vi "AnalogAQ Canales.vi"(8 "error in":errorcluster, 9 "Numero de Muestras":i32=1000, 10 "Frecuencia":dbl=1000.0 format="%0.2f", 11 "Canales":tag[](array[tag])) -> (0 "error out":errorcluster, 3 "Classic DAQmx Task Name":refnum<k21>)   [LabVIEW 2020]
uses:
  <vilib>/DAQmx/create/channels.llb/DAQmx Create Channel (AI-Voltage-Basic).vi
  <vilib>/DAQmx/configure/timing.llb/DAQmx Timing (Sample Clock).vi
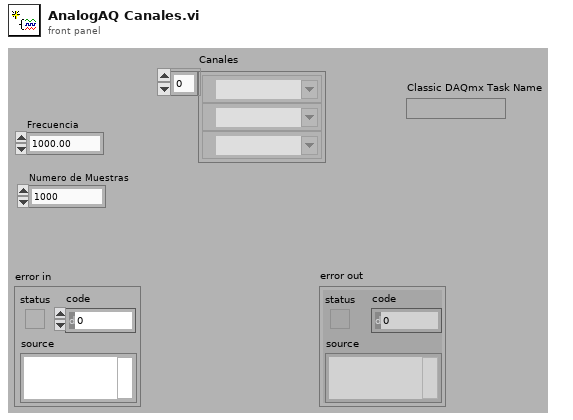
[diagram p1: front panel]
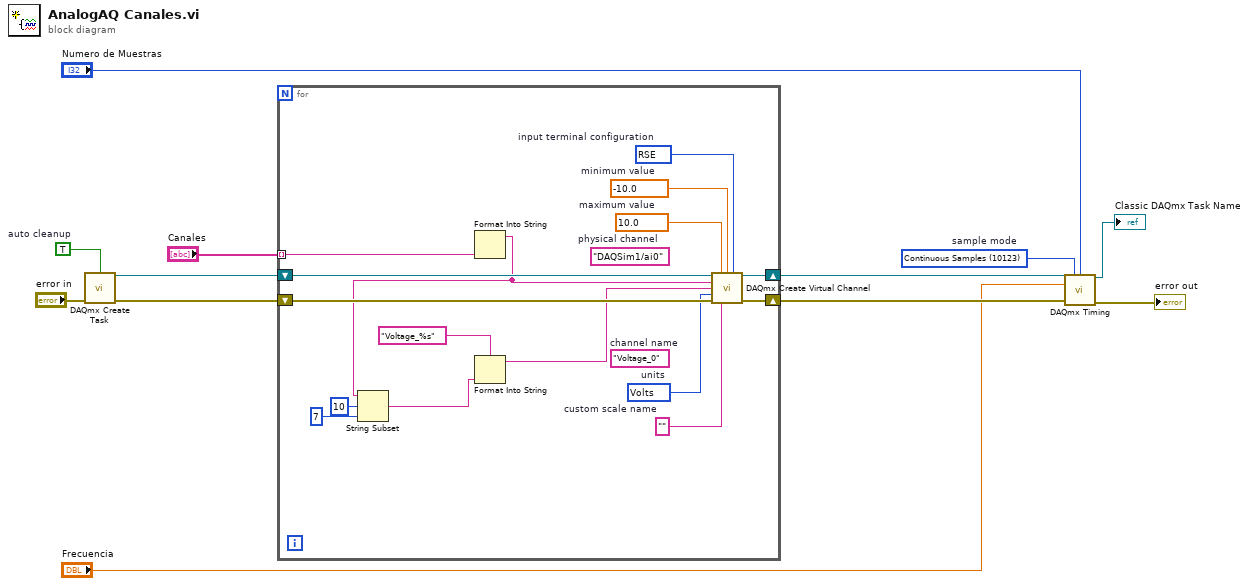
[diagram p0: block diagram]
diagram:
  w5 = 10123 items=["Finite Samples"=10178, "Continuous Samples"=10123, "Hardware Timed Single Point"=12522]  # sample mode
  w10 = TRUE  # auto cleanup
  n1 = call <vilib>:"DAQmx Create Task.vi"("auto cleanup"=w10, "error in"="error in") -> ("task out"=w9:refnum<k21>, "error out"=w11:errorcluster)  [unwired: 12 in]
  n2 = for {
    shift-right: [w23] -> w8
    shift-left: w11 -> [w28]
    shift-right: [w20] -> w7
    shift-left: w9 -> [w27]
    tunnel: "Canales" -> [w17] mode=indexing
    w21 = 10083 items=["default"=-1, "RSE"=10083, "NRSE"=10078, "Differential"=10106, "Pseudodifferential"=12529]  # input terminal configuration
    w22 = 10348 items=["Volts"=10348, "From Custom Scale"=10065]  # units
    (unwired) "Voltage_0"  # channel name
    w24 = ""  # custom scale name
    w25 = -10.0  # minimum value
    w26 = 10.0  # maximum value
    (unwired) "DAQSim1/ai0"  # physical channel
    n3 = Format Into String(w17) -> (resulting string=w16:string)  [unwired: 3 in, 1 out]
    n4 = String Subset(string=w16, offset (0)=10, length (rest)=7 ("length (rest)")) -> (substring=w13:string)
    n5 = Format Into String(format string="Voltage_%s", w13) -> (resulting string=w18:string)  [unwired: 2 in, 1 out]
    n6 = call-poly <vilib>:"DAQmx Create Virtual Channel.vi"("task in"=w27, "maximum value"=w26, "minimum value"=w25, "input terminal configuration"=w21, "physical channels"=w16, "name to assign"=w18, "units"=w22, "error in"=w28, "custom scale name"=w24) -> ("task out"=w20:refnum<k21>, "error out"=w23:errorcluster)  [unwired: 5 in]
  }
  n7 = call-poly <vilib>:"DAQmx Timing.vi"("task/channels in"=w7, "sample mode"=w5, "samples per channel"="Numero de Muestras", "rate"="Frecuencia", "error in"=w8) -> ("task out"=→"Classic DAQmx Task Name":refnum<k21>, "error out"=→"error out":errorcluster)  [unwired: 9 in]
